vi "Que_Insert.vi"(6 "TimeOut(-1)":i32=-1, 8 "error in":errorcluster, 9 "Data":variant, 10 "Event":string, 11 "QueueName":string) -> (0 "error out":errorcluster, 1 "timed out?":bool)   [LabVIEW 2016]
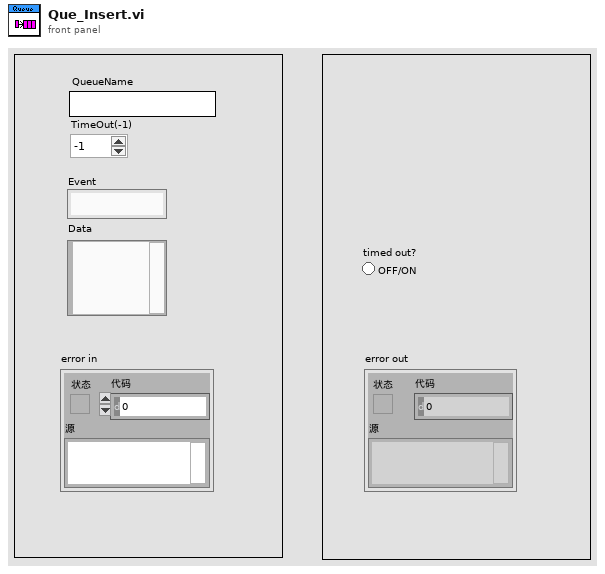
[diagram p1: front panel]
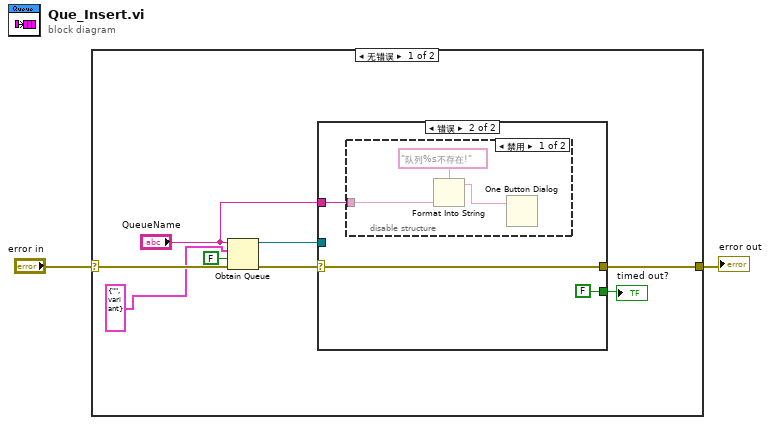
[diagram p0: block diagram]
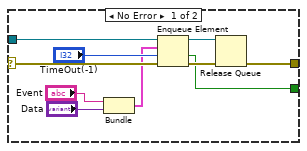
[diagram p2: hidden frame]
diagram:
  n1 = case shown="无错误" "error in" {
    selector: "error in" -> [w5 w27]
    tunnel: [w6 w27] -> w2
    frame No Error {
      n2 = Obtain Queue(name (unnamed)="QueueName", element data type=cluster{string, "变体":variant} {"", "变体"=variant}, create if not found? (T)=FALSE ("如未找到是否创建？(T)"), error in (no error)=w5) -> (queue out=w8:refnum<queue>, error out=w9:errorcluster)  [unwired: 1 in, 1 out]
      n3 = case shown="错误" w9 {
        selector: w9 -> [w20 w22]
        tunnel: w8 -> [w19 _]
        tunnel: [w13 w22] -> w6
        tunnel: [w12 FALSE ("timed out?")] -> w7
        tunnel: "QueueName" -> [_ w21]
        frame No Error {
          n4 = Bundle("Event"="Event", "Data"="Data") -> (w11:cluster{"Event":string, "Data":variant})  [unwired: 1 in]
          n5 = Enqueue Element(queue=w19, element=w11, timeout in ms (-1)="TimeOut(-1)", error in (no error)=w20) -> (queue out=w15:refnum<queue>, timed out?=w12:bool, error out=w16:errorcluster)
          n6 = Release Queue(queue=w15, error in (no error)=w16) -> (error out=w13:errorcluster)  [unwired: 1 in, 2 out]
        }
        frame Error {
          n7 = disable-structure shown="禁用" {
            disable-tunnel: w21 -> [w26 _]
            frame Disabled {
              n8 = Format Into String(format string="队列%s不存在!" ("格式字符串"), w26) -> (resulting string=w25:string)  [unwired: 2 in, 1 out]
              n9 = One Button Dialog(message=w25) -> ()  [unwired: 1 in, 1 out]
            }
            frame Enabled {
            }
          }
        }
      }
      "timed out?" <- w7
    }
    frame Error {
    }
  }
  "error out" <- w2
